vi "cycle_inflation_attempt3.vi"() -> ()   [LabVIEW 2014]
doc: "This VI demonstrates the individual configuration of settings in I/W, W/I, and continuous operation modes.\n\nThis VI is not meant to be used with infusion-only models. \n\nNotes:\n(1) If continuous mode is selected, infuse volumes/rates will be used."
uses:
  <instrlib>/KD Scientific 2XX Series/KD Scientific 2XX Series.lvlib
panel:
  in  "number of steps":i32
  out "Units":string
  out "Delivered Volume":dbl
  in  "stop":bool
  out "Status":T1
  in  "Baud Rate (9600)":u32(ring)=9600 items=["300"=300, "1200"=1200, "2400"=2400, "4800"=4800, "9600"=9600]
  in  "Withdrawal Settings":T2={"Flow Rate (5)"=5.0, "Volume (10)"=10.0, "Volume Units (ml)"=enum."milliliters (ml)", "Rate Units (ml/min.)"=enum."milliliters per minute (ml/min.)"} {"Volume (10)" format="%#.3g"}
  in  "Diameter (8.75 mm)":dbl=8.75
  in  "Infusion Settings":T2={"Flow Rate (5)"=5.0, "Volume (10)"=10.0, "Volume Units (ml)"=enum."milliliters (ml)", "Rate Units (ml/min.)"=enum."milliliters per minute (ml/min.)"}
  in  "Address (0)":i32 format="%0.0f"
  in  "error in (no error)":errorcluster
  in  "VISA resource name":refnum<visa-resource-name>="COM1"
  # "© 2005 National Instruments Corporation.  ALL RIGHTS RESERVED."
  # "RS-232 Settings"
  # "General Settings"
  # "Pump Status"
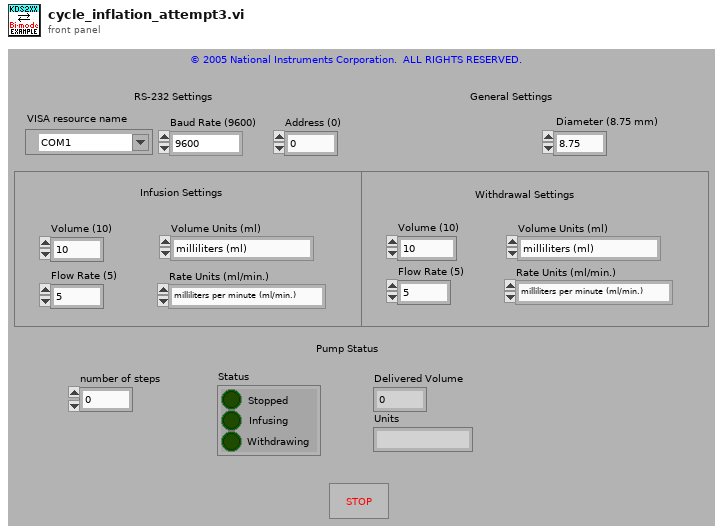
[diagram p1: front panel]
types:
  T1 = cluster{"Stopped":bool, "Infusing":bool, "Withdrawing":bool}
  T2 = cluster{"Flow Rate (5)":dbl, "Volume (10)":dbl, "Volume Units (ml)":enum16{"milliliters (ml)", "microliters (ul)"}, "Rate Units (ml/min.)":enum16{"milliliters per minute (ml/min.)", "milliliters per hour (ml/hr.)", "microliters per minute (ul/min.)", "microliters per hour (ul/hr.)"}}
  T3 = enum16{"milliliters per minute (ml/min.)", "milliliters per hour (ml/hr.)", "microliters per minute (ul/min.)", "microliters per hour (ul/hr.)"}
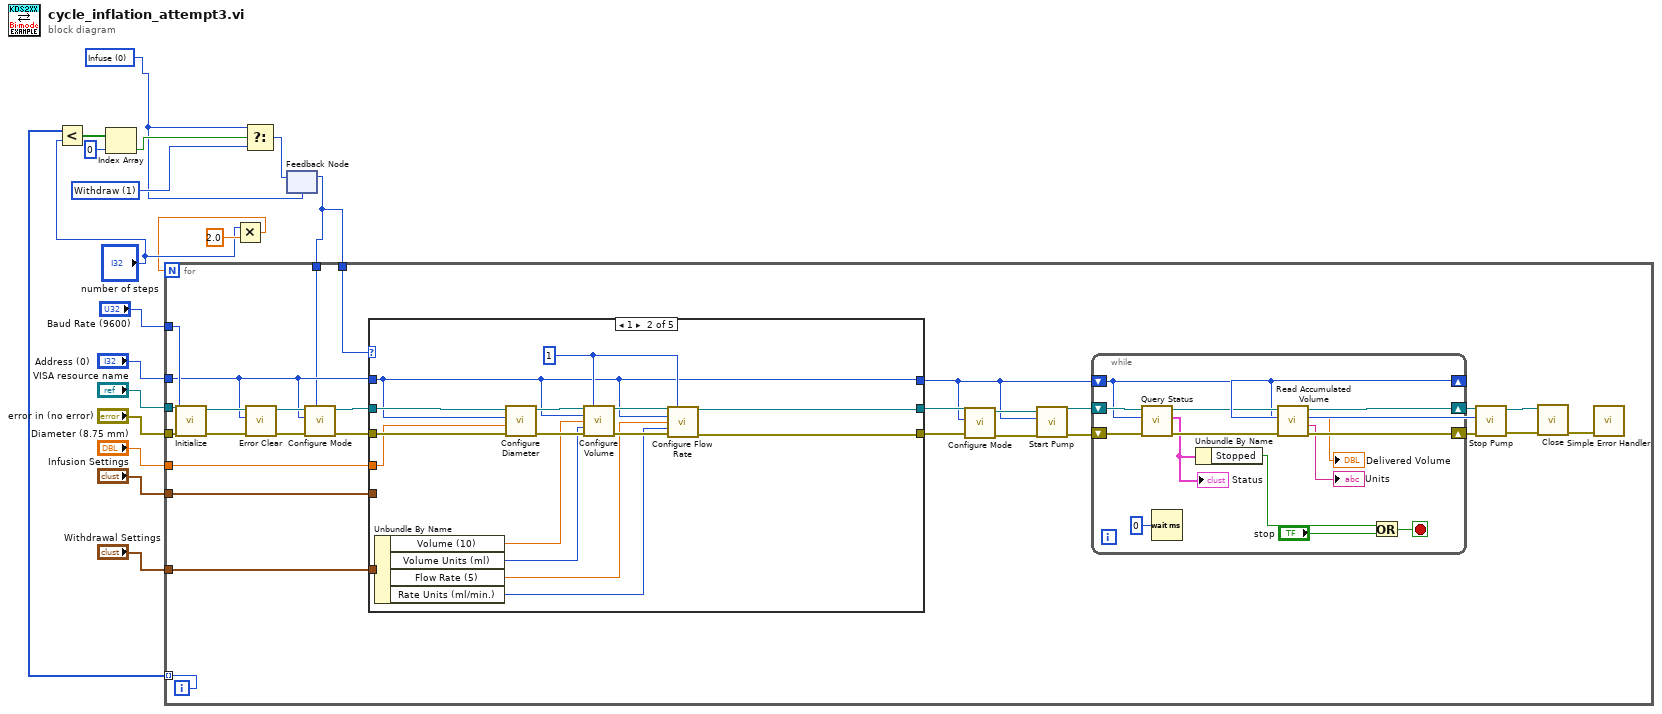
[diagram p0: block diagram]
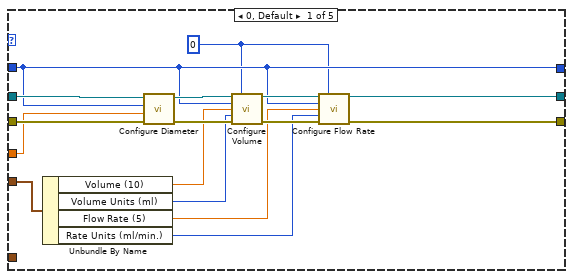
[diagram p2: hidden frame]
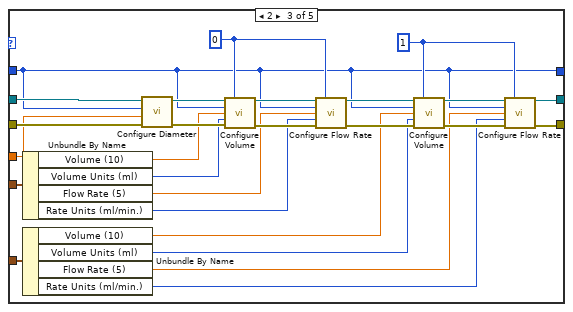
[diagram p3: hidden frame]
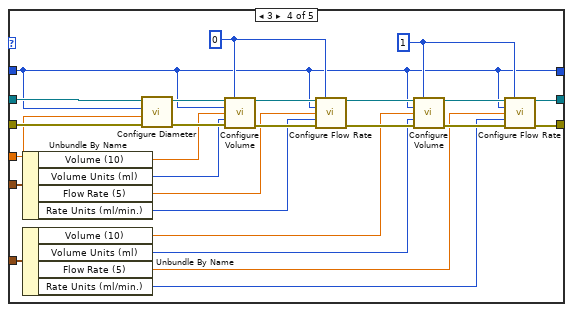
[diagram p4: hidden frame]
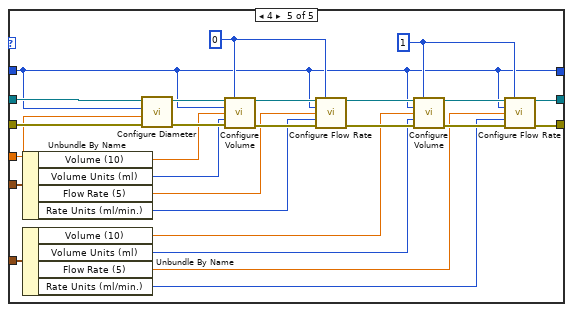
[diagram p5: hidden frame]
diagram:
  w11 = u16 1 items=["Withdraw"=1]
  w5 = u16 0 items=["Infuse"] ("Mode (infuse)")
  n1 = Multiply(x="number of steps", y=2.0) -> (x*y=w1:dbl)
  n2 = feedback #1(w5) -> (w4:u16)
  n3 = for {
    N: w1 -> [_]
    tunnel: "VISA resource name" -> [w47]
    tunnel: "error in (no error)" -> [w46]
    tunnel: "Infusion Settings" -> [w41]
    tunnel: "Withdrawal Settings" -> [w40]
    tunnel: "Diameter (8.75 mm)" -> [w39]
    tunnel: "Baud Rate (9600)" -> [w34]
    tunnel: "Address (0)" -> [w22]
    tunnel: [w21] -> w10 mode=indexing
    tunnel: w4 -> [w20]
    tunnel: w4 -> [w19]
    i -> [w21]
    n4 = call <instrlib>:"Initialize.vi"("error in (no error)"=w46, "Baud Rate (9600)"=w34, "VISA resource name"=w47) -> ("error out"=w24:errorcluster, "VISA resource name out"=w23:refnum<visa-resource-name>)  [unwired: 7 in]
    n5 = call <instrlib>:"Error Clear.vi"("error in (no error)"=w24, "Address (0)"=w22, "VISA resource name"=w23) -> ("error out"=w25:errorcluster, "VISA resource name out"=w26:refnum<visa-resource-name>)  [unwired: 6 in, 1 out]
    n6 = call <instrlib>:"Configure Mode.vi"("Mode (infuse)"=w20, "error in (no error)"=w25, "Address (0)"=w22, "VISA resource name"=w26) -> ("error out"=w28:errorcluster, "VISA resource name out"=w27:refnum<visa-resource-name>)  [unwired: 6 in]
    n7 = case shown="1" w19 {
      tunnel: w41 -> [w57 _ w105 w131 w157]
      tunnel: w40 -> [_ w79 w104 w130 w156]
      tunnel: w27 -> [w63 w78 w103 w129 w155]
      tunnel: w28 -> [w62 w74 w102 w128 w154]
      tunnel: w39 -> [w56 w70 w85 w111 w137]
      tunnel: [w55 w64 w80 w106 w132] -> w29
      tunnel: w22 -> [w55 w64 w80 w106 w132]
      tunnel: [w50 w75 w82 w108 w134] -> w33
      tunnel: [w49 w71 w81 w107 w133] -> w32
      frame 0, Default {
        w48 = 0
        n8 = Unbundle By Name(w57) -> ("Volume (10)"=w54:dbl, "Volume Units (ml)"=w53:enum16{"milliliters (ml)", "microliters (ul)"}, "Flow Rate (5)"=w52:dbl, "Rate Units (ml/min.)"=w51:T3)
        n9 = call <instrlib>:"Configure Diameter.vi"("error in (no error)"=w62, "Diameter (8.75 mm)"=w56, "Address (0)"=w55, "VISA resource name"=w63) -> ("error out"=w60:errorcluster, "VISA resource name out"=w61:refnum<visa-resource-name>)  [unwired: 6 in]
        n10 = call <instrlib>:"Configure Volume.vi"("VISA resource name"=w61, "Mode (infuse)"=w48, "Address (0)"=w55, "Volume (100)"=w54, "Units (0: milliliters)"=w53, "error in (no error)"=w60) -> ("VISA resource name out"=w59:refnum<visa-resource-name>, "error out"=w58:errorcluster)  [unwired: 8 in]
        n11 = call <instrlib>:"Configure Flow Rate.vi"("VISA resource name"=w59, "Mode (infuse)"=w48, "Address (0)"=w55, "Flow Rate (5)"=w52, "Units (0: milliliters per minute)"=w51, "error in (no error)"=w58) -> ("VISA resource name out"=w50:refnum<visa-resource-name>, "error out"=w49:errorcluster)  [unwired: 8 in]
      }
      frame 1 {
        w65 = 1
        n12 = Unbundle By Name(w79) -> ("Volume (10)"=w69:dbl, "Volume Units (ml)"=w68:enum16{"milliliters (ml)", "microliters (ul)"}, "Flow Rate (5)"=w67:dbl, "Rate Units (ml/min.)"=w66:T3)
        n13 = call <instrlib>:"Configure Diameter.vi"("error in (no error)"=w74, "Diameter (8.75 mm)"=w70, "Address (0)"=w64, "VISA resource name"=w78) -> ("error out"=w73:errorcluster, "VISA resource name out"=w77:refnum<visa-resource-name>)  [unwired: 6 in]
        n14 = call <instrlib>:"Configure Volume.vi"("VISA resource name"=w77, "Mode (infuse)"=w65, "Address (0)"=w64, "Volume (100)"=w69, "Units (0: milliliters)"=w68, "error in (no error)"=w73) -> ("VISA resource name out"=w76:refnum<visa-resource-name>, "error out"=w72:errorcluster)  [unwired: 8 in]
        n15 = call <instrlib>:"Configure Flow Rate.vi"("VISA resource name"=w76, "Mode (infuse)"=w65, "Address (0)"=w64, "Flow Rate (5)"=w67, "Units (0: milliliters per minute)"=w66, "error in (no error)"=w72) -> ("VISA resource name out"=w75:refnum<visa-resource-name>, "error out"=w71:errorcluster)  [unwired: 8 in]
      }
      frame 2 {
        w83 = 1
        w84 = 0
        n16 = Unbundle By Name(w105) -> ("Volume (10)"=w93:dbl, "Volume Units (ml)"=w92:enum16{"milliliters (ml)", "microliters (ul)"}, "Flow Rate (5)"=w91:dbl, "Rate Units (ml/min.)"=w90:T3)
        n17 = Unbundle By Name(w104) -> ("Volume (10)"=w89:dbl, "Volume Units (ml)"=w88:enum16{"milliliters (ml)", "microliters (ul)"}, "Flow Rate (5)"=w87:dbl, "Rate Units (ml/min.)"=w86:T3)
        n18 = call <instrlib>:"Configure Diameter.vi"("error in (no error)"=w102, "Diameter (8.75 mm)"=w85, "Address (0)"=w80, "VISA resource name"=w103) -> ("error out"=w97:errorcluster, "VISA resource name out"=w101:refnum<visa-resource-name>)  [unwired: 6 in]
        n19 = call <instrlib>:"Configure Volume.vi"("VISA resource name"=w101, "Mode (infuse)"=w84, "Address (0)"=w80, "Volume (100)"=w93, "Units (0: milliliters)"=w92, "error in (no error)"=w97) -> ("VISA resource name out"=w100:refnum<visa-resource-name>, "error out"=w96:errorcluster)  [unwired: 8 in]
        n20 = call <instrlib>:"Configure Flow Rate.vi"("VISA resource name"=w100, "Mode (infuse)"=w84, "Address (0)"=w80, "Flow Rate (5)"=w91, "Units (0: milliliters per minute)"=w90, "error in (no error)"=w96) -> ("VISA resource name out"=w99:refnum<visa-resource-name>, "error out"=w95:errorcluster)  [unwired: 8 in]
        n21 = call <instrlib>:"Configure Volume.vi"("VISA resource name"=w99, "Mode (infuse)"=w83, "Address (0)"=w80, "Volume (100)"=w89, "Units (0: milliliters)"=w88, "error in (no error)"=w95) -> ("VISA resource name out"=w98:refnum<visa-resource-name>, "error out"=w94:errorcluster)  [unwired: 8 in]
        n22 = call <instrlib>:"Configure Flow Rate.vi"("VISA resource name"=w98, "Mode (infuse)"=w83, "Address (0)"=w80, "Flow Rate (5)"=w87, "Units (0: milliliters per minute)"=w86, "error in (no error)"=w94) -> ("VISA resource name out"=w82:refnum<visa-resource-name>, "error out"=w81:errorcluster)  [unwired: 8 in]
      }
      frame 3 {
        w109 = 1
        w110 = 0
        n23 = Unbundle By Name(w131) -> ("Volume (10)"=w119:dbl, "Volume Units (ml)"=w118:enum16{"milliliters (ml)", "microliters (ul)"}, "Flow Rate (5)"=w117:dbl, "Rate Units (ml/min.)"=w116:T3)
        n24 = Unbundle By Name(w130) -> ("Volume (10)"=w115:dbl, "Volume Units (ml)"=w114:enum16{"milliliters (ml)", "microliters (ul)"}, "Flow Rate (5)"=w113:dbl, "Rate Units (ml/min.)"=w112:T3)
        n25 = call <instrlib>:"Configure Diameter.vi"("error in (no error)"=w128, "Diameter (8.75 mm)"=w111, "Address (0)"=w106, "VISA resource name"=w129) -> ("error out"=w123:errorcluster, "VISA resource name out"=w127:refnum<visa-resource-name>)  [unwired: 6 in]
        n26 = call <instrlib>:"Configure Volume.vi"("VISA resource name"=w127, "Mode (infuse)"=w110, "Address (0)"=w106, "Volume (100)"=w119, "Units (0: milliliters)"=w118, "error in (no error)"=w123) -> ("VISA resource name out"=w126:refnum<visa-resource-name>, "error out"=w122:errorcluster)  [unwired: 8 in]
        n27 = call <instrlib>:"Configure Flow Rate.vi"("VISA resource name"=w126, "Mode (infuse)"=w110, "Address (0)"=w106, "Flow Rate (5)"=w117, "Units (0: milliliters per minute)"=w116, "error in (no error)"=w122) -> ("VISA resource name out"=w125:refnum<visa-resource-name>, "error out"=w121:errorcluster)  [unwired: 8 in]
        n28 = call <instrlib>:"Configure Volume.vi"("VISA resource name"=w125, "Mode (infuse)"=w109, "Address (0)"=w106, "Volume (100)"=w115, "Units (0: milliliters)"=w114, "error in (no error)"=w121) -> ("VISA resource name out"=w124:refnum<visa-resource-name>, "error out"=w120:errorcluster)  [unwired: 8 in]
        n29 = call <instrlib>:"Configure Flow Rate.vi"("VISA resource name"=w124, "Mode (infuse)"=w109, "Address (0)"=w106, "Flow Rate (5)"=w113, "Units (0: milliliters per minute)"=w112, "error in (no error)"=w120) -> ("VISA resource name out"=w108:refnum<visa-resource-name>, "error out"=w107:errorcluster)  [unwired: 8 in]
      }
      frame 4 {
        w135 = 1
        w136 = 0
        n30 = Unbundle By Name(w157) -> ("Volume (10)"=w145:dbl, "Volume Units (ml)"=w144:enum16{"milliliters (ml)", "microliters (ul)"}, "Flow Rate (5)"=w143:dbl, "Rate Units (ml/min.)"=w142:T3)
        n31 = Unbundle By Name(w156) -> ("Volume (10)"=w141:dbl, "Volume Units (ml)"=w140:enum16{"milliliters (ml)", "microliters (ul)"}, "Flow Rate (5)"=w139:dbl, "Rate Units (ml/min.)"=w138:T3)
        n32 = call <instrlib>:"Configure Diameter.vi"("error in (no error)"=w154, "Diameter (8.75 mm)"=w137, "Address (0)"=w132, "VISA resource name"=w155) -> ("error out"=w149:errorcluster, "VISA resource name out"=w153:refnum<visa-resource-name>)  [unwired: 6 in]
        n33 = call <instrlib>:"Configure Volume.vi"("VISA resource name"=w153, "Mode (infuse)"=w136, "Address (0)"=w132, "Volume (100)"=w145, "Units (0: milliliters)"=w144, "error in (no error)"=w149) -> ("VISA resource name out"=w152:refnum<visa-resource-name>, "error out"=w148:errorcluster)  [unwired: 8 in]
        n34 = call <instrlib>:"Configure Flow Rate.vi"("VISA resource name"=w152, "Mode (infuse)"=w136, "Address (0)"=w132, "Flow Rate (5)"=w143, "Units (0: milliliters per minute)"=w142, "error in (no error)"=w148) -> ("VISA resource name out"=w151:refnum<visa-resource-name>, "error out"=w147:errorcluster)  [unwired: 8 in]
        n35 = call <instrlib>:"Configure Volume.vi"("VISA resource name"=w151, "Mode (infuse)"=w135, "Address (0)"=w132, "Volume (100)"=w141, "Units (0: milliliters)"=w140, "error in (no error)"=w147) -> ("VISA resource name out"=w150:refnum<visa-resource-name>, "error out"=w146:errorcluster)  [unwired: 8 in]
        n36 = call <instrlib>:"Configure Flow Rate.vi"("VISA resource name"=w150, "Mode (infuse)"=w135, "Address (0)"=w132, "Flow Rate (5)"=w139, "Units (0: milliliters per minute)"=w138, "error in (no error)"=w146) -> ("VISA resource name out"=w134:refnum<visa-resource-name>, "error out"=w133:errorcluster)  [unwired: 8 in]
      }
    }
    n37 = call <instrlib>:"Configure Mode.vi"("error in (no error)"=w32, "Address (0)"=w29, "VISA resource name"=w33) -> ("error out"=w30:errorcluster, "VISA resource name out"=w31:refnum<visa-resource-name>)  [unwired: 7 in]
    n38 = call <instrlib>:"Start Pump.vi"("error in (no error)"=w30, "Address (0)"=w29, "VISA resource name"=w31) -> ("error out"=w44:errorcluster, "VISA resource name out"=w45:refnum<visa-resource-name>)  [unwired: 7 in]
    n39 = while {
      shift-right: [w160] -> w38
      shift-left: w29 -> [w160]
      shift-right: [w162] -> w43
      shift-left: w45 -> [w168]
      shift-right: [w161] -> w42
      shift-left: w44 -> [w169]
      stop <- w166 stop-if-true
      n40 = call <instrlib>:"Query Status.vi"("error in (no error)"=w169, "Address (0)"=w160, "VISA resource name"=w168) -> ("error out"=w171:errorcluster, "Status"=w167:T1, "VISA resource name out"=w163:refnum<visa-resource-name>)  [unwired: 6 in]
      "Status" <- w167
      n41 = Wait (ms)(milliseconds to wait=u32 0) -> ()  [unwired: 1 out]
      n42 = Unbundle By Name(w167) -> ("Stopped"=w165:bool)
      n43 = call <instrlib>:"Read Accumulated Volume.vi"("error in (no error)"=w171, "Address (0)"=w160, "VISA resource name"=w163) -> ("error out"=w161:errorcluster, "Units"=→"Units":string, "Delivered Volume"=→"Delivered Volume":dbl, "VISA resource name out"=w162:refnum<visa-resource-name>)  [unwired: 5 in]
      n44 = Or(x=w165, y="stop") -> (x .or. y?=w166:bool)
    }
    n45 = call <instrlib>:"Stop Pump.vi"("error in (no error)"=w42, "Address (0)"=w38, "VISA resource name"=w43) -> ("error out"=w36:errorcluster, "VISA resource name out"=w35:refnum<visa-resource-name>)  [unwired: 7 in]
    n46 = call <instrlib>:"Close.vi"("error in (no error)"=w36, "VISA resource name"=w35) -> ("error out"=w37:errorcluster)  [unwired: 9 in]
    n47 = call <vilib>:"Simple Error Handler.vi"("error in (no error)"=w37) -> ()  [unwired: 4 in, 5 out]
  }
  n48 = Less?(x=w10, y="number of steps") -> (x < y?=w9:bool[])
  n49 = Index Array(array=w9, index=0) -> (element=w7:bool)
  n50 = Select(t=w5, s=w7, f=w11) -> (s? t:f=w6:u16)
  n51 = feedback-in #1(w6) -> ()
